vi "readFromXML.vi"(8 "error in (no error)":errorcluster, 10 "XMLin":string, 11 "WavefrontTargetConfiguration in":refnum<class "WavefrontTargetConfiguration.lvclass">) -> (0 "error out":errorcluster, 3 "WavefrontTargetConfiguration out":refnum<class "WavefrontTargetConfiguration.lvclass">)   [LabVIEW 2022 SP3, in "TCSDataDefinitions.lvlib" / "TCSCommand.lvlib" / "TargetConfiguration.lvlib" / "WavefrontTargetConfiguration.lvclass"]
uses:
  WavefrontTargetConfiguration.lvclass
  TargetConfiguration/TargetConfiguration.lvclass
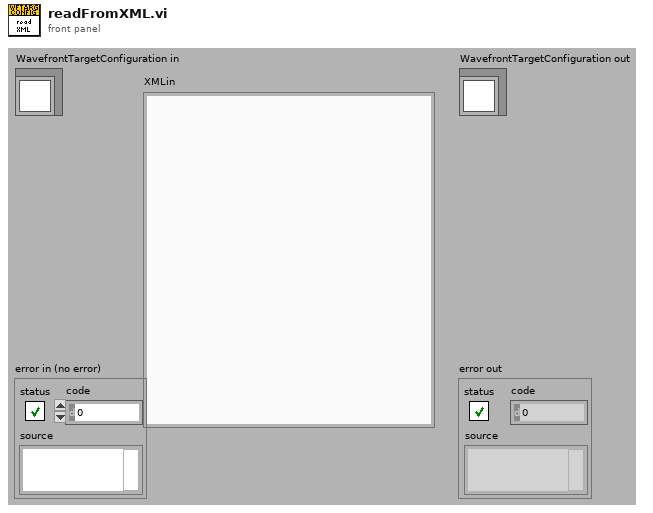
[diagram p1: front panel]
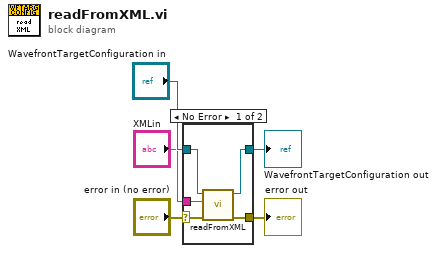
[diagram p0: block diagram]
diagram:
  n1 = case shown="No Error" "error in (no error)" {
    selector: "error in (no error)" -> [w7 w12]
    tunnel: [w6 w12] -> w4
    tunnel: [w9 w11] -> w2
    tunnel: "WavefrontTargetConfiguration in" -> [w10 w11]
    tunnel: "XMLin" -> [w8 _]
    frame No Error {
      n2 = call-parent "readFromXML.vi"("error in (no error)"=w7, "XMLin"=w8, "TargetConfiguration in"=w10) -> ("error out"=w6:errorcluster, "TargetConfiguration out"=w9:refnum<class "WavefrontTargetConfiguration.lvclass">)  [unwired: 7 in]
    }
    frame Error {
    }
  }
  "error out" <- w4
  "WavefrontTargetConfiguration out" <- w2
